vi "Mes Remote Telephone.vi"(8 "error in (no error)":errorcluster, 11 "Main":T1={"Tite"="", "Base path"=path "", "Table"=[], "Stations"=[], "Shield Array"=[], "UPHs"=[], "VISA"={"VISA"="", "baud rate"=9600, "data bits"=8, "parity"=enum."None", "stop bits"=10, "flow control"=0}, "Path"={"roof"=path "", "Config"=path "", "Png"=path ""}, "Ctr"={"DB Dispaly"=refnum, "Error Table"=refnum, "Display"=refnum, "Login"=refnum, "Exit"=refnum, "FTT_Submit"=refnum}, "Login"={"User"="", "Grade"=""}, "information"={"cause"="", "Type"=enum."Inform", "code"=0, "Suroce"="", "Status"=FALSE}, "Local DB"={"Connstr"="", "Database"={"Constr"={"Driver"="", "Server"="", "User"="", "Pwd"="", "Database"=""}, "conn ref"=refnum, "State"=FALSE}}, "Remote DB"={"Connstr"="", "Database"={"Constr"={"Driver"="", "Server"="", "User"="", "Pwd"="", "Database"=""}, "conn ref"=refnum, "State"=FALSE}}, "FTT TV"="", "ExchangeTime"=0, "NVH"="", "EOL Path"=path ""} {"VISA"."flow control" items=["None", "XON/XOFF", "RTS/CTS", "XON/XOFF & RTS/CTS", "DTR/DSR", "XON/XOFF & DTR/DSR"]; "VISA"."stop bits" items=["1.0"=10, "1.5"=15, "2.0"=20]}) -> (0 "error out":errorcluster)   [LabVIEW 2014]
uses:
  Type'def/Mes Table.ctl
  <vilib>/ptbypt/NI_PtbyPt.lvlib
  Type'def/UPH Config.ctl
  VISA/Ctr/VISA Ctr.ctl
  Type'def/Main Ctr Ref.ctl
  Type'def/User Login.ctl
  Database/Ctr/Constr.ctl
  <vilib>/addons/database/Connection.llb/Conn ObjectReference.ctl
  <vilib>/addons/database/NI_Database_API.lvlib
  Database/Ctr/Conneect State.ctl
  Type'def/MainCtr.ctl
panel:
  in  "x 2":bool
  out "数组":i32[](array[numeric])
  in  "x":bool
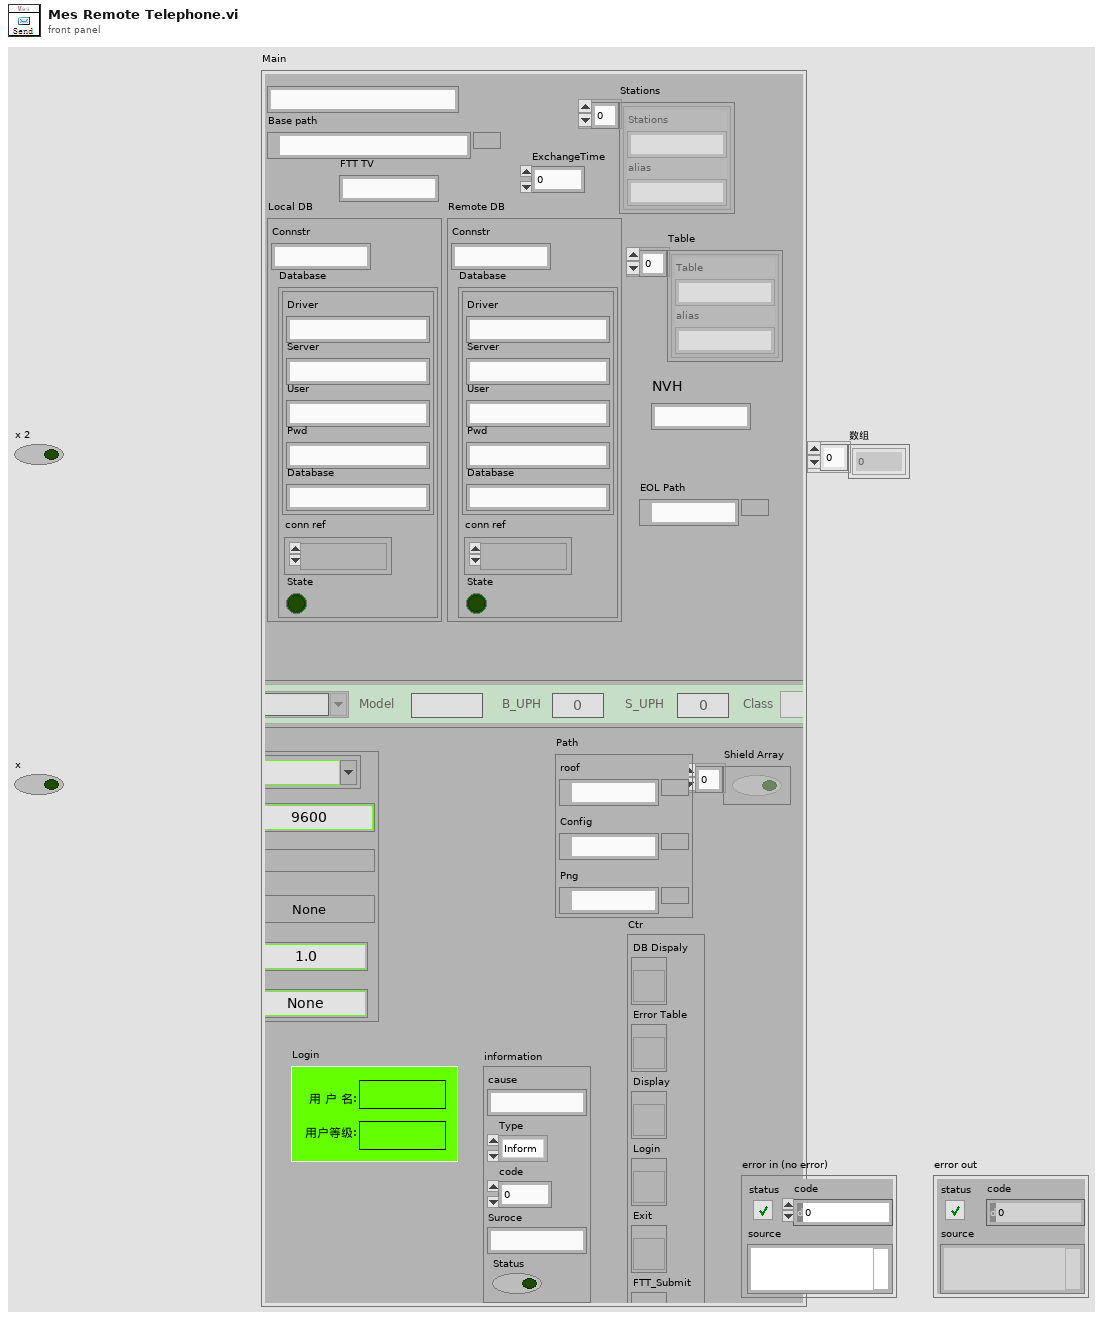
[diagram p1: front panel]
types:
  T1 = typedef "MainCtr.ctl" = cluster{"Tite":string, "Base path":path, "Table":cluster{"Table":string, "alias":string}[], "Stations":cluster{"Stations":string, "alias":string}[], "Shield Array":bool[], "UPHs":T2[], "VISA":T3, "Path":cluster{"roof":path, "Config":path, "Png":path}, "Ctr":T4, "Login":T5, "information":cluster{"cause":string, "Type":enum16{"Inform", "Warning", "Alarm"}, "code":i32, "Suroce":string, "Status":bool}, "Local DB":cluster{"Connstr":string, "Database":T6}, "Remote DB":cluster{"Connstr":string, "Database":T6}, "FTT TV":string, "ExchangeTime":i32, "NVH":string, "EOL Path":path}
  T2 = typedef "UPH Config.ctl" = cluster{"Line_No":string, "Model":string, "B_UPH ":i16, "S_UPH  ":i16, "Class":enum16{"Big", "Small"}}
  T3 = typedef "VISA Ctr.ctl" = cluster{"VISA":refnum<visa-resource-name>, "baud rate":u32, "data bits":u16, "parity":enum16{"None", "Odd", "Even", "Mark", "Space"}, "stop bits":u16, "flow control":u16}
  T4 = typedef "Main Ctr Ref.ctl" = cluster{"DB Dispaly":refnum<vi>, "Error Table":refnum<vi>, "Display":refnum<vi>, "Login":refnum<vi>, "Exit":refnum<vi>, "FTT_Submit":refnum<vi>}
  T5 = typedef "User Login.ctl" = cluster{"User":string, "Grade":string}
  T6 = typedef "Conneect State.ctl" = cluster{"Constr":T7, "conn ref":T8, "State":bool}
  T7 = typedef "Constr.ctl" = cluster{"Driver":string, "Server":string, "User":string, "Pwd":string, "Database":string}
  T8 = typedef "NI_Database_API.lvlib/Conn ObjectReference.ctl" = refnum<k1>
  T9 = cluster{"Model":string, "Actual":string, "NG":string}
  T10 = cluster{"cause":string, "Type":enum16{"Inform", "Warning", "Alarm"}, "code":i32, "Suroce":string, "Status":bool}
  T11 = typedef "Mes Table.ctl" = cluster{"DateInfo":timestamp, "Shift":string, "Line_Name":string, "ProjectName":string, "AvaType":string, "AvaValue":string, "Remark":string}
  T12 = cluster{"Outline_Type":string[], "Mess FTT":cluster{"Model":string, "Actual":string, "NG":string}, "Model":string[], "Main ":T1, "mes":T11, "information":cluster{"cause":string, "Type":enum16{"Inform", "Warning", "Alarm"}, "code":i32, "Suroce":string, "Status":bool}, "Insert/Update(Run)":bool[], "CT":string, "Mode":enum16{"Eight", "EModel", "Outline"}, "Insert/Update(History)":bool[]}
  T13 = typedef "FTT Display Type.ctl" = cluster{"Line.No":string, "Model":string, "Color":string, "UPH":dbl, "Plan":dbl, "Target Rate":dbl, "Target ":dbl, "Actual":dbl, "FTT":dbl, "FTT Rate":dbl, "Repaired":dbl, "Reject":dbl, "Ouline":dbl, "Line State":string}
  T14 = cluster{"Display":T13, "Class":enum16{"Big", "Small"}}
  T15 = typedef "Phone Var.ctl" = cluster{"Mes":bool, "Model":string}
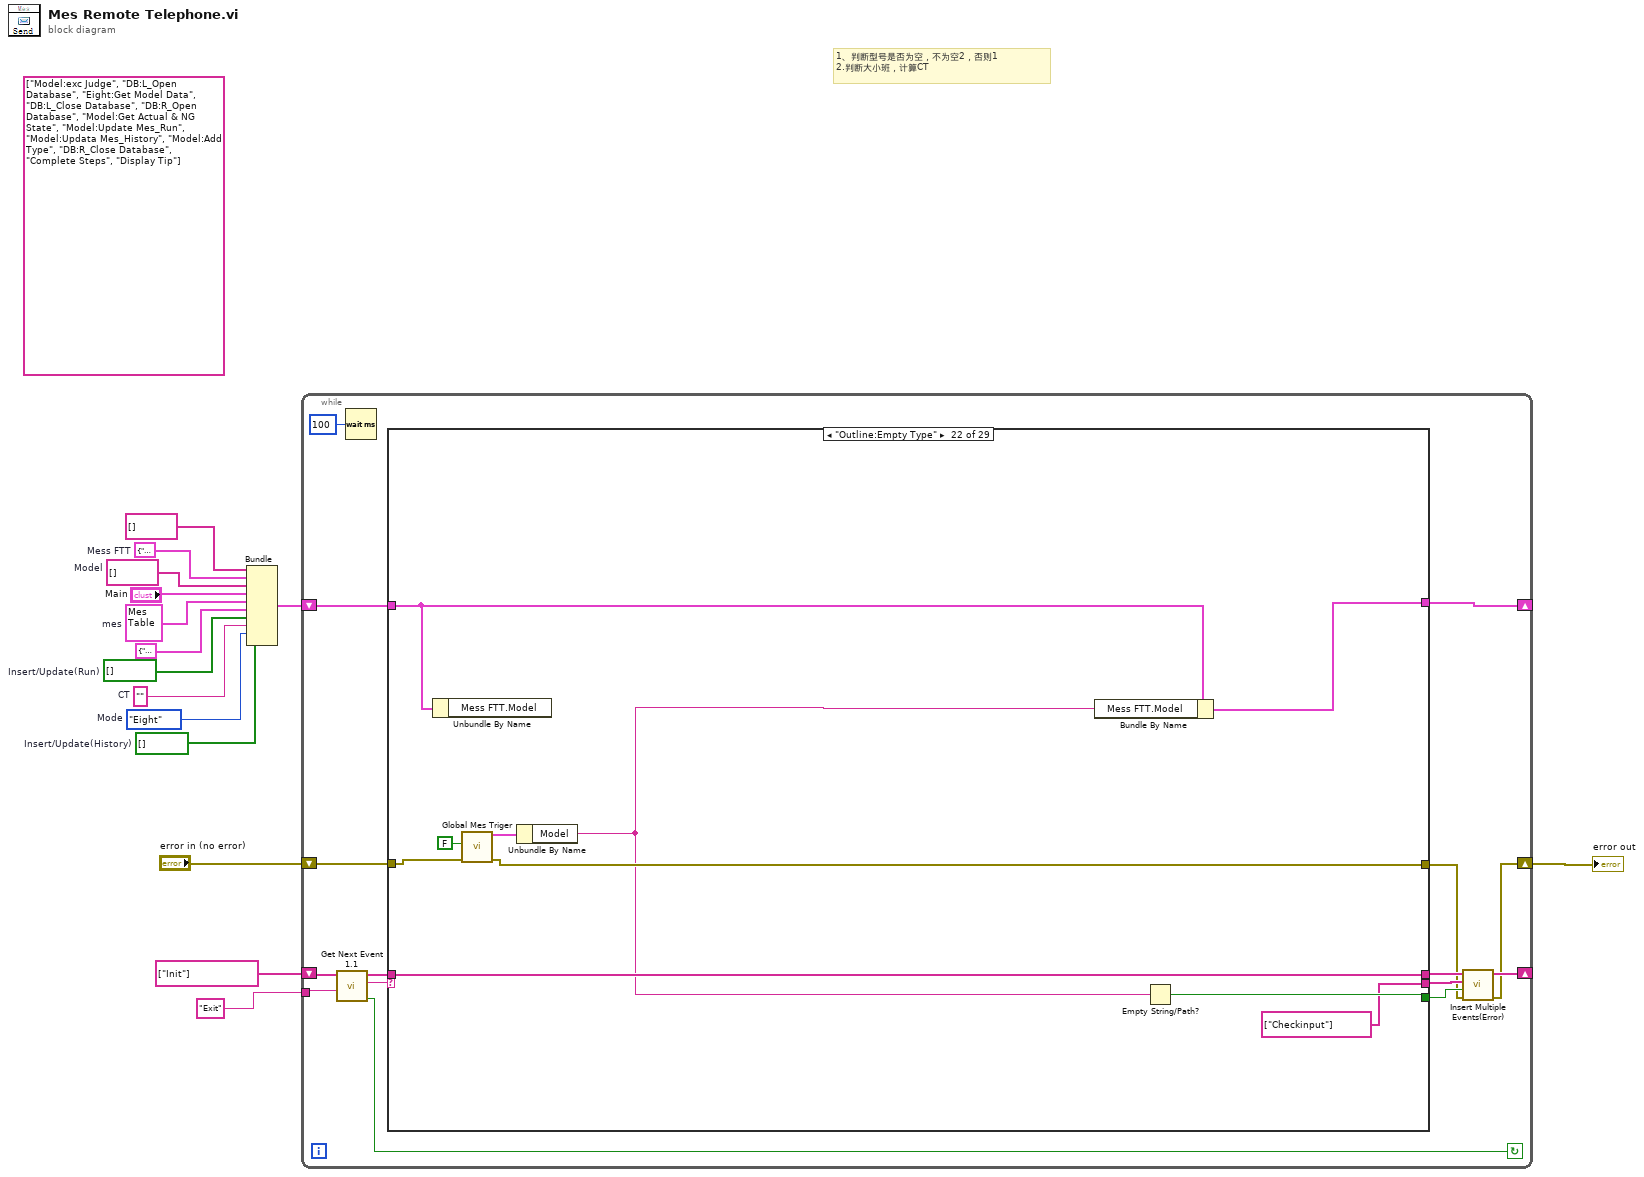
[diagram p0: block diagram]
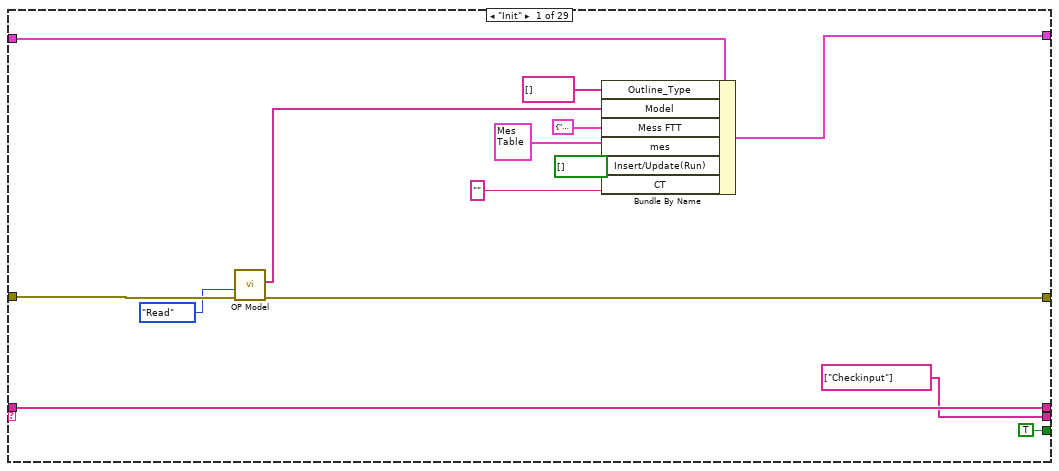
[diagram p2: hidden frame]
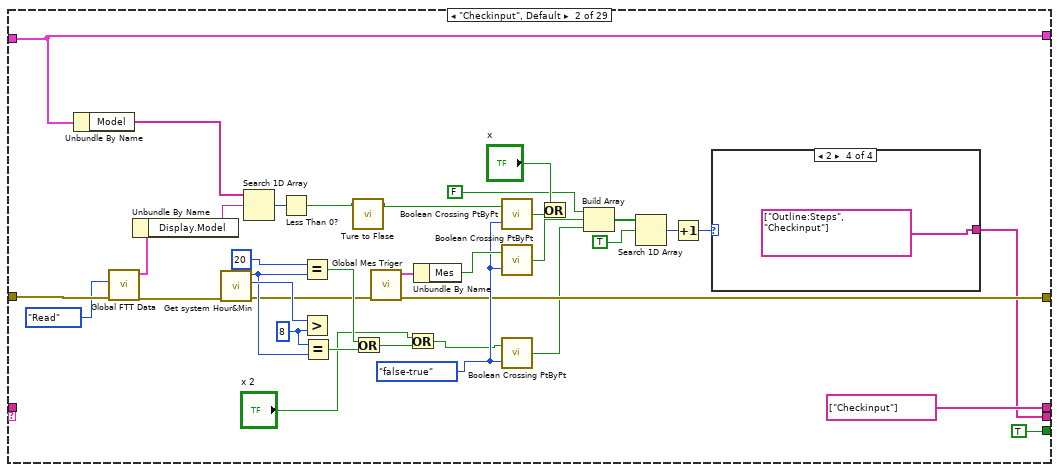
[diagram p3: hidden frame]
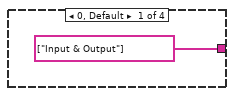
[diagram p4: hidden frame]
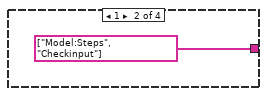
[diagram p5: hidden frame]
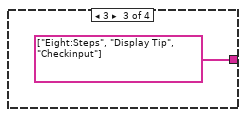
[diagram p6: hidden frame]
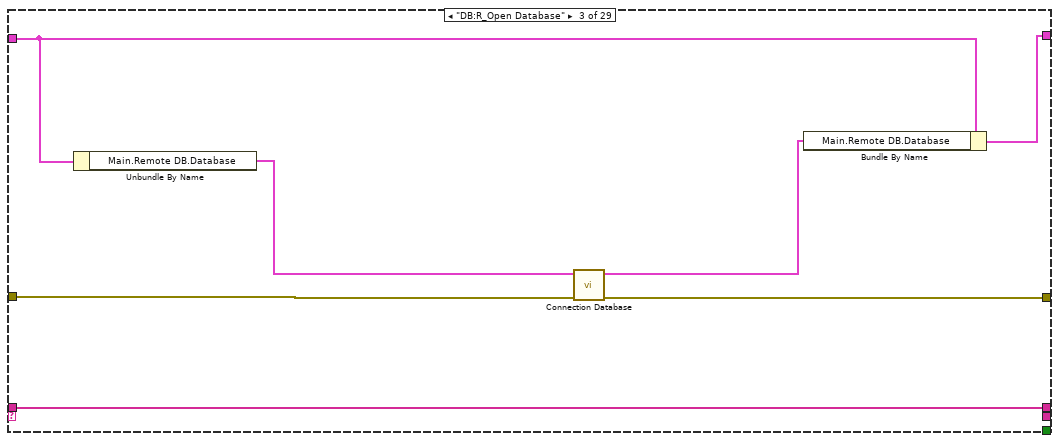
[diagram p7: hidden frame]
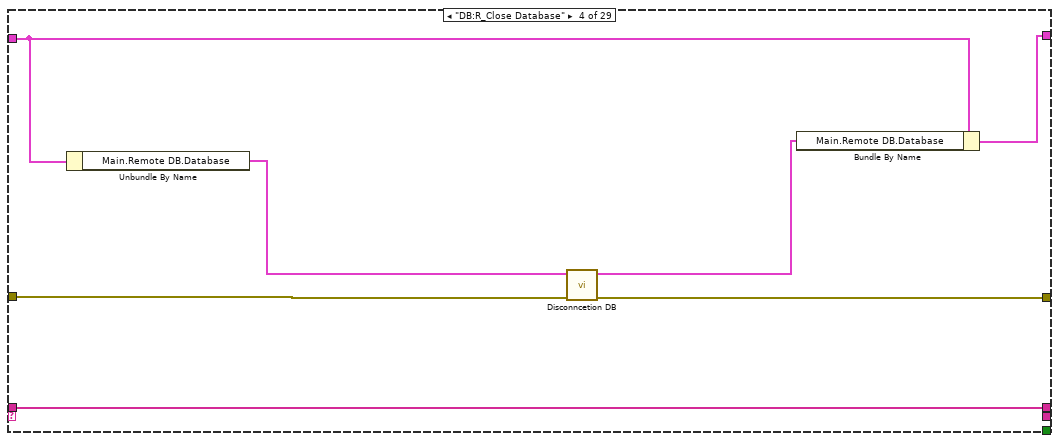
[diagram p8: hidden frame]
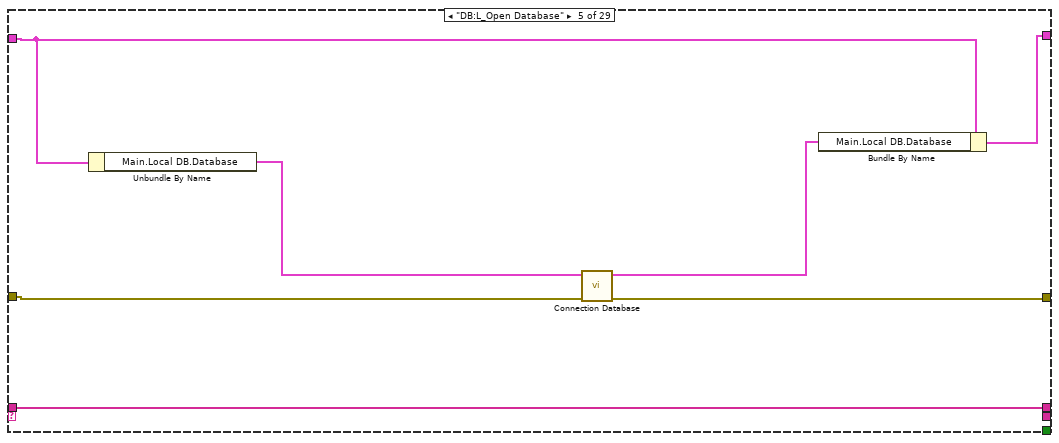
[diagram p9: hidden frame]
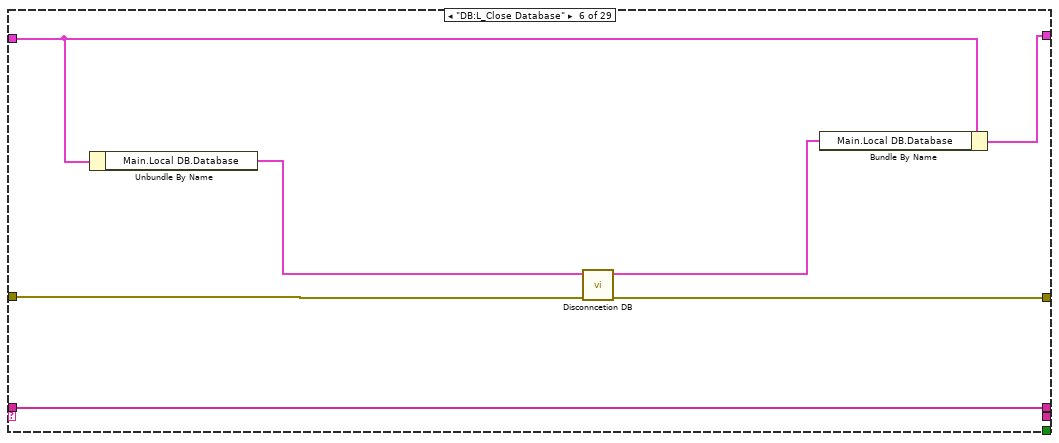
[diagram p10: hidden frame]
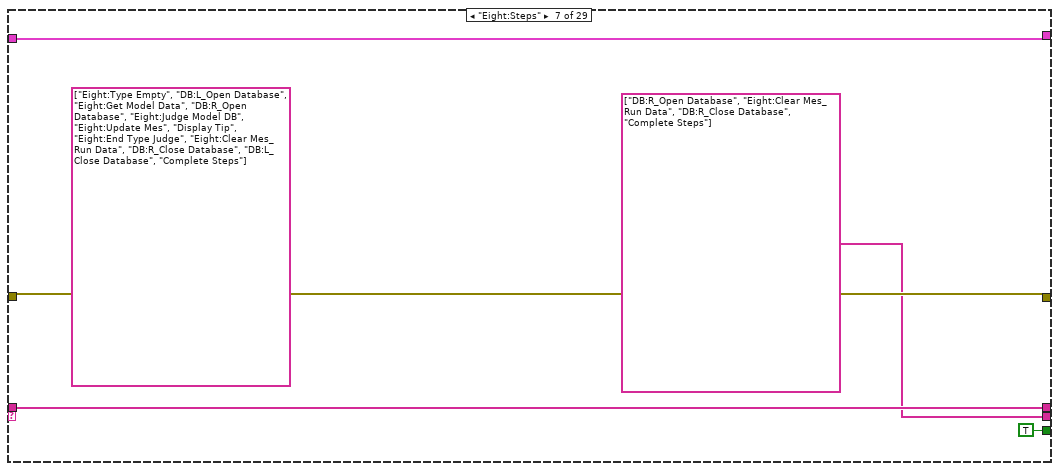
[diagram p11: hidden frame]
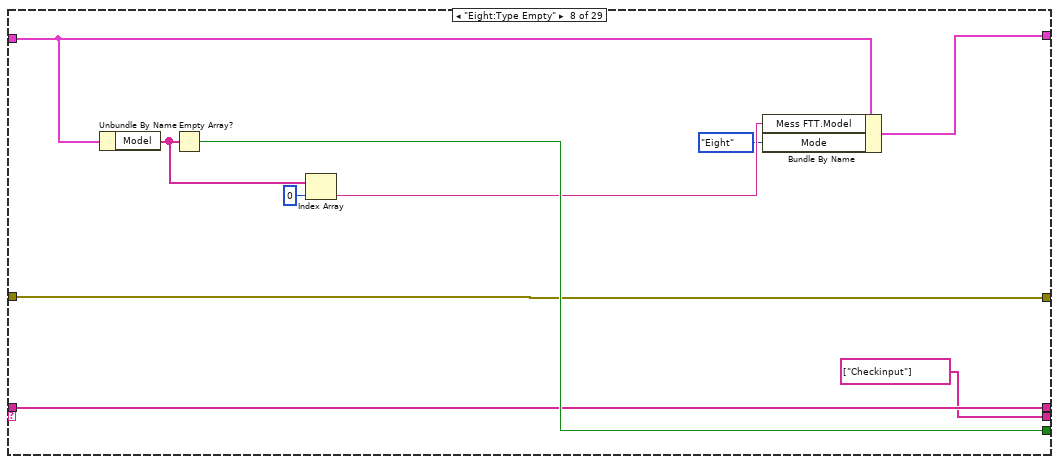
[diagram p12: hidden frame]
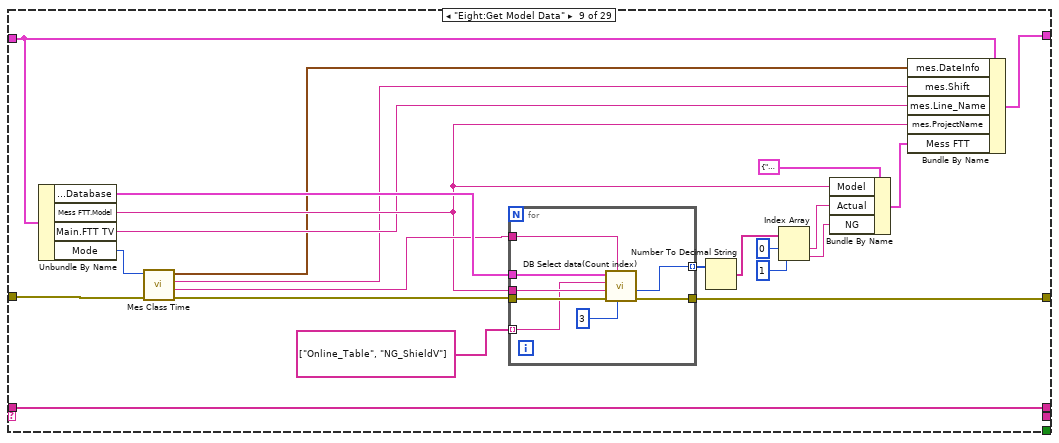
[diagram p13: hidden frame]
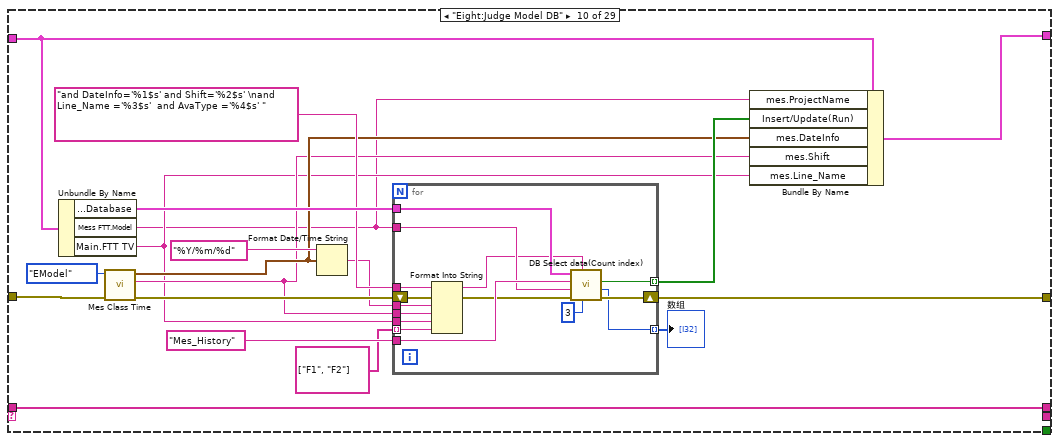
[diagram p14: hidden frame]
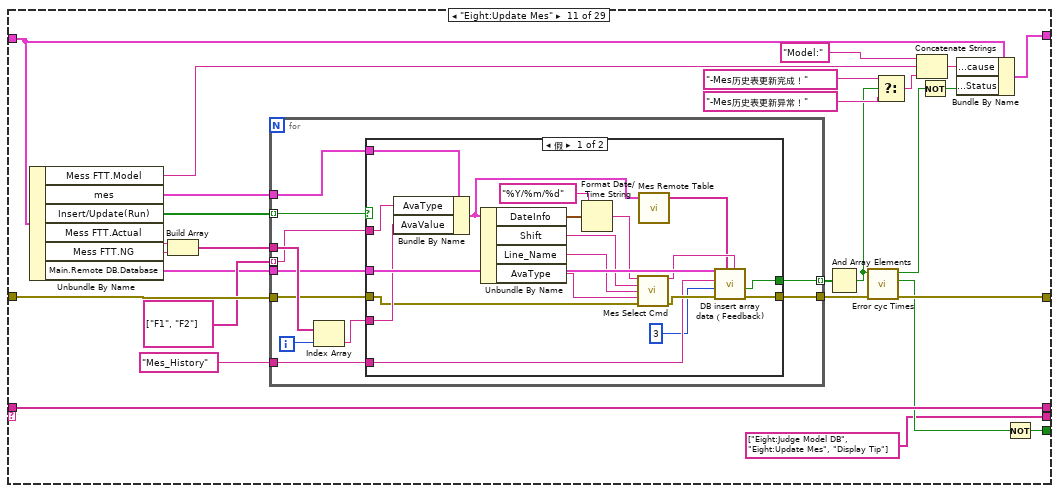
[diagram p15: hidden frame]
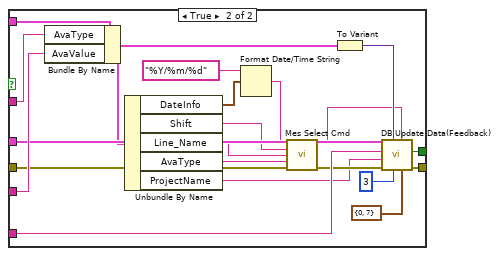
[diagram p16: hidden frame]
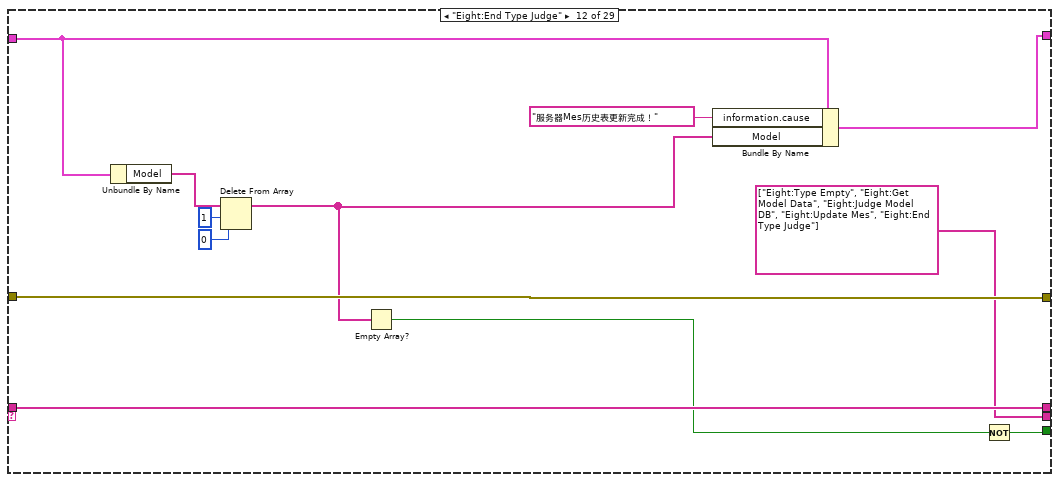
[diagram p17: hidden frame]
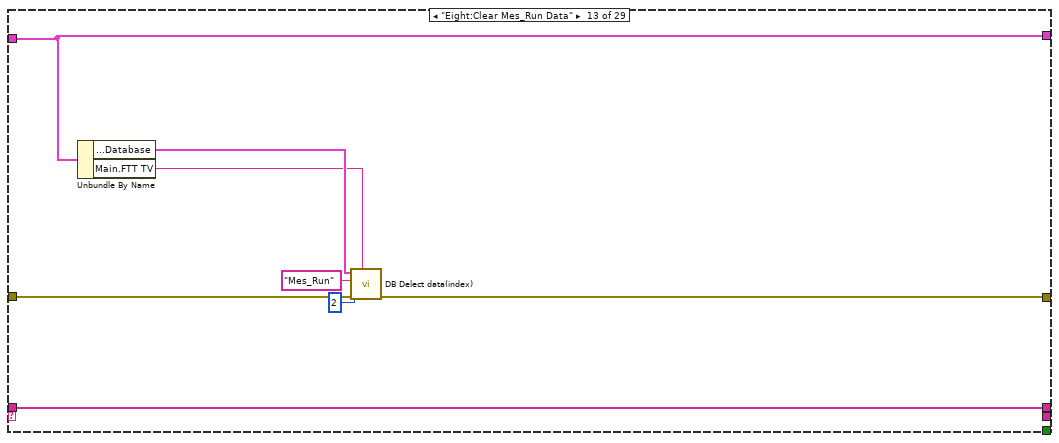
[diagram p18: hidden frame]
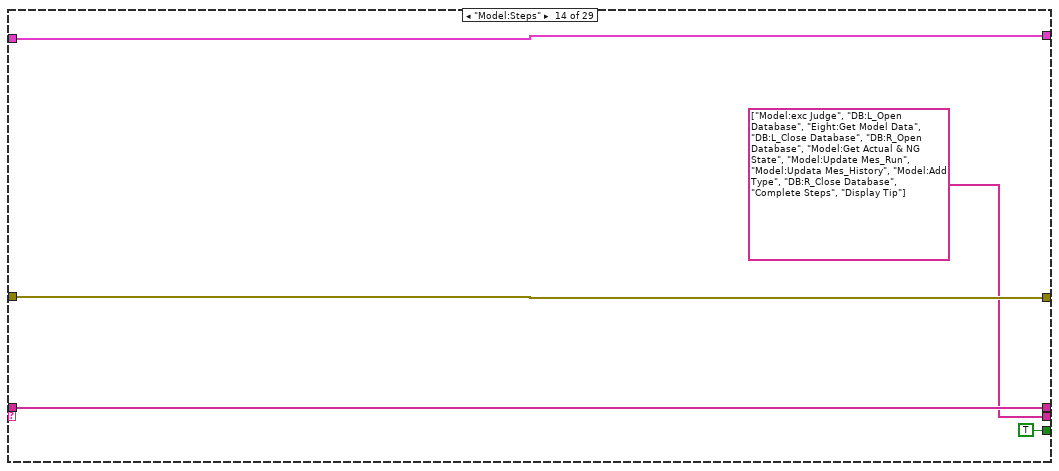
[diagram p19: hidden frame]
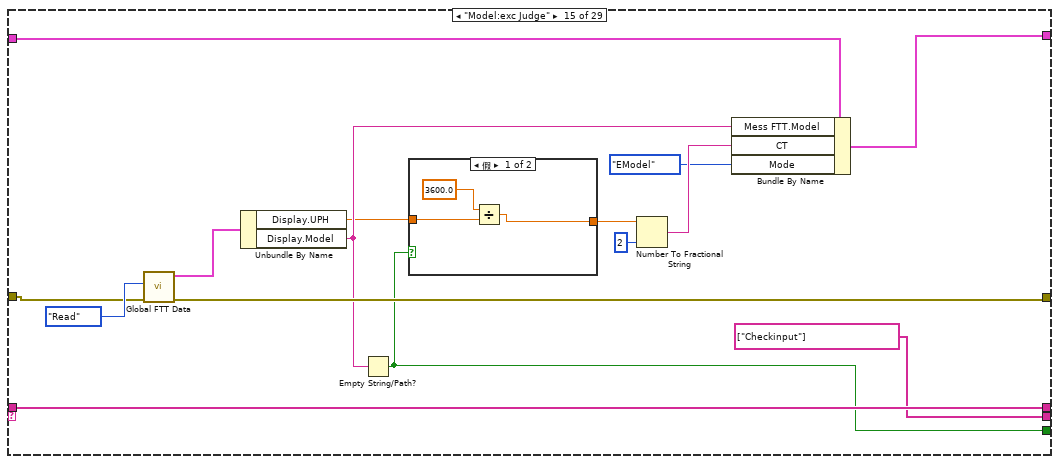
[diagram p20: hidden frame]
diagram:
  w1 = bool[] []  # Insert/Update(History)
  (unwired) string[] ["Model:exc Judge", "DB:L_Open Database", "Eight:Get Model Data", "DB:L_Close Database", "DB:R_Open Database", "Model:Get Actual & NG State", "Model:Update Mes_Run", "Model:Updata Mes_History", "Model:Add Type", "DB:R_Close Database", "Complete Steps", "Display Tip"]
  w2 = enum16{"Eight", "EModel", "Outline"}."Eight"  # Mode
  w3 = ""  # CT
  w5 = bool[] []  # Insert/Update(Run)
  w6 = T9 {"Model"="", "Actual"="", "NG"=""}  # Mess FTT
  w7 = string[] []  # Model
  w10 = T11 {"DateInfo"=timestamp(0 s since 1904-01-01), "Shift"="", "Line_Name"="", "ProjectName"="", "AvaType"="", "AvaValue"="", "Remark"=""}  # mes
  # "1、判断型号是否为空，不为空2，否则1\n2.判断大小班，计算CT"
  n1 = Bundle("Outline_Type"=string[] [], "Mess FTT"=w6, "Model"=w7, "Main"="Main", "mes"=w10, "information"=T10 {"cause"="", "Type"=enum."Inform", "code"=0, "Suroce"="", "Status"=FALSE}, "Insert/Update(Run)"=w5, "CT"=w3, "Mode"=w2, "Insert/Update(History)"=w1) -> (w12:T12)  [unwired: 1 in]
  n2 = while {
    tunnel: "Exit" ("Exit Event") -> [w27]
    shift-right: [w23] -> _
    shift-left: string[] ["Init"] -> [w28]
    shift-right: [w16] -> w9
    shift-left: "error in (no error)" -> [w26]
    shift-right: [w19] -> _
    shift-left: w12 -> [w24]
    stop <- w29 continue-if-true
    n3 = call "Get Next Event 1.1.vi"("Exit Event"=w27, "event queue in"=w28) -> ("Condition (Exit:F)"=w29:bool, "next event"=w30:string, "event queue out"=w25:string[])  [unwired: 6 in, 1 out]
    n4 = Wait (ms)(milliseconds to wait=u32 100) -> ()  [unwired: 1 out]
    n5 = case shown="\"Outline:Empty Type\"" w30 {
      tunnel: w26 -> [w34 w78 w89 w97 w103 w110 w114 w126 w135 w173 w217 w276 w288 w293 w308 w324 w349 w391 w463 w542 w561 w572 w585 w668 w673 w680 w686 w689 w697]
      tunnel: w25 -> [w44 _ w85 w98 w100 w106 w116 w125 w149 w176 w218 w275 w282 w292 w306 w322 w346 w389 w485 w553 w567 w577 w583 w661 w672 w681 w685 w692 w700]
      tunnel: w24 -> [w35 w60 w87 w94 w102 w109 w117 w123 w138 w165 w203 w278 w289 w294 w305 w321 w350 w388 w462 w552 w565 w574 w584 w663 w675 w682 w687 w693 w704]
      tunnel: [w33 w61 w86 w96 w101 w107 w114 w126 w146 w168 w206 w276 w283 w293 w307 w323 w348 w390 w483 w541 w559 w571 w582 w668 w673 w676 w686 w694 w705] -> w17
      tunnel: [w44 string[] ["Checkinput"] w85 w98 w100 w106 w116 w125 w149 w176 w218 w275 w282 w292 w306 w322 w346 w389 w485 w553 w567 w577 w583 w661 w672 w681 w685 w692 w700] -> w22
      tunnel: [TRUE ("Insert all? (T)") TRUE ("Insert all? (T)") _ _ _ _ TRUE ("Insert all? (T)") w127 _ _ w205 w273 _ TRUE ("Insert all? (T)") w300 _ _ w385 w484 _ TRUE ("Insert all? (T)") w576 w579 w658 _ w678 TRUE ("Insert all? (T)") _ TRUE ("Insert all? (T)")] -> w21
      tunnel: [string[] ["Checkinput"] w53 _ _ _ _ string[] ["DB:R_Open Database", "Eight:Clear Mes_Run Data", "DB:R_Close Database", "Complete Steps"] string[] ["Checkinput"] _ _ string[] ["Eight:Judge Model DB", "Eight:Update Mes", "Display Tip"] string[] ["Eight:Type Empty", "Eight:Get Model Data", "Eight:Judge Model DB", "Eight:Update Mes", "Eight:End Type Judge"] _ string[] ["Model:exc Judge", "DB:L_Open Database", "Eight:Get Model Data", "DB:L_Close Database", "DB:R_Open Database", "Model:Get Actual & NG State", "Model:Update Mes_Run", "Model:Updata Mes_History", "Model:Add Type", "DB:R_Close Database", "Complete Steps", "Display Tip"] string[] ["Checkinput"] _ _ w378 w475 _ string[] ["Model:exc Judge", "Outline:Empty Type", "DB:L_Open Database", "Eight:Get Model Data", "DB:R_Open Database", "Model:Get Actual & NG State(Run)", "Model:Get Actual & NG State(History)", "Model:Update Mes_Run", "Model:Updata Mes_History", "DB:L_Close Database", "DB:R_Close Database", "Display Tip "] string[] ["Checkinput"] string[] ["Outline:Mes_Run Update"] string[] ["Outline:Empty Type", "Eight:Get Model Data", "Outline:Mes_Run Update", "Outline:End Type Judge"] _ string[] ["Quit"] string[] ["Exit"] _ string[] ["Checkinput"]] -> w20
      tunnel: [w36 w60 w88 w93 w99 w108 w117 w122 w137 w164 w202 w277 w289 w294 w304 w320 w347 w387 w480 w551 w564 w573 w586 w662 w674 w682 w687 w693 w704] -> w19
      frame "Init" {
        n6 = call "OP Model.vi"("error in (no error)"=w34, "Enum"=enum16{"init", "Read", "Write"}."Read") -> ("error out"=w33:errorcluster, "ArrayStr out"=w31:string[])  [unwired: 7 in, 1 out]
        n7 = Bundle By Name(cluster=w35, "Outline_Type"=string[] [], "Model"=w31, "Mess FTT"=T9 {"Model"="", "Actual"="", "NG"=""}, "mes"=T11 {"DateInfo"=timestamp(0 s since 1904-01-01), "Shift"="", "Line_Name"="", "ProjectName"="", "AvaType"="", "AvaValue"="", "Remark"=""}, "Insert/Update(Run)"=bool[] [] ("Insert/Update"), "CT"="") -> (w36:T12)
      }
      frame "Checkinput", Default {
        w62 = enum16{"either", "false-true", "true-false"}."false-true" ("direction")
        w70 = 8 ("y")
        n8 = Unbundle By Name(w60) -> ("Model"=w74:string[])
        n9 = call "Global FTT Data.vi"("error in (no error)"=w78, "Mode"=enum16{"Read", "Write"}."Read") -> ("error out"=w72:errorcluster, "Cluster"=w76:T14)  [unwired: 8 in]
        n10 = Unbundle By Name(w76) -> ("Display.Model"=w75:string)
        n11 = call "Get system Hour&Min.vi"("error in (no error)"=w72) -> ("error out"=w65:errorcluster, "minute"=w69:i32, "hour"=w68:i32)  [unwired: 7 in, 1 out]
        n12 = Search 1D Array(1D array=w74, element=w75) -> (index of element=w73:i32)  [unwired: 1 in]
        n13 = Less Than 0?(x=w73) -> (x < 0?=w50:bool)
        n14 = Equal?(x=20, y=w68) -> (x = y?=w66:bool)
        n15 = Greater?(x=w69, y=w70) -> ()  [unwired: 1 out]
        n16 = Equal?(x=w70, y=w68) -> (x = y?=w67:bool)
        n17 = call "Ture to Flase.vi"("in"=w50) -> ("Out"=w49:bool)  [unwired: 4 in]
        n18 = Or(x=w66, y=w67) -> (x .or. y?=w48:bool)
        n19 = call "Global Mes Triger.vi"("error in (no error)"=w65) -> ("error out"=w61:errorcluster, "Var out"=w64:T15)  [unwired: 9 in]
        n20 = Or(x="x 2", y=w48) -> (x .or. y?=w47:bool)
        n21 = Unbundle By Name(w64) -> ("Mes"=w63:bool)
        n22 = call <vilib>:"Boolean Crossing PtByPt.vi"("direction"=w62, "input"=w49) -> ("crossing"=w52:bool)  [unwired: 1 in]
        n23 = call <vilib>:"Boolean Crossing PtByPt.vi"("direction"=w62, "input"=w63) -> ("crossing"=w59:bool)  [unwired: 1 in]
        n24 = call <vilib>:"Boolean Crossing PtByPt.vi"("direction"=w62, "input"=w47) -> ("crossing"=w58:bool)  [unwired: 1 in]
        n25 = Or(x="x", y=w52) -> ()  [unwired: 1 out]
        n26 = Build Array(FALSE ("element"), w59, w58) -> (w57:bool[])
        n27 = Search 1D Array(1D array=w57, element=TRUE) -> (index of element=w55:i32)  [unwired: 1 in]
        n28 = Increment(x=w55) -> (x+1=w54:i32)
        n29 = case shown="2" w54 {
          tunnel: [string[] ["Input & Output"] string[] ["Model:Steps", "Checkinput"] string[] ["Eight:Steps", "Display Tip", "Checkinput"] string[] ["Outline:Steps", "Checkinput"]] -> w53
          frame 0, Default {
          }
          frame 1 {
          }
          frame 3 {
          }
          frame 2 {
          }
        }
      }
      frame "DB:R_Open Database" {
        n30 = Unbundle By Name(w87) -> ("Main.Remote DB.Database"=w91:T6)
        n31 = call "Connection Database.vi"("error in (no error)"=w89, "Connncet State"=w91) -> ("error out"=w86:errorcluster, "Connncet State out"=w90:T6)  [unwired: 8 in]
        n32 = Bundle By Name(cluster=w87, "Main.Remote DB.Database"=w90) -> (w88:T12)
      }
      frame "DB:R_Close Database" {
        n33 = Unbundle By Name(w94) -> ("Main.Remote DB.Database"=w95:T6)
        n34 = call "Disconncetion DB.vi"("error in (no error)"=w97, "Connncet State"=w95) -> ("error out"=w96:errorcluster, "Connect State"=w92:T6)  [unwired: 8 in]
        n35 = Bundle By Name(cluster=w94, "Main.Remote DB.Database"=w92) -> (w93:T12)
      }
      frame "DB:L_Open Database" {
        n36 = Unbundle By Name(w102) -> ("Main.Local DB.Database"=w105:T6)
        n37 = call "Connection Database.vi"("error in (no error)"=w103, "Connncet State"=w105) -> ("error out"=w101:errorcluster, "Connncet State out"=w104:T6)  [unwired: 8 in]
        n38 = Bundle By Name(cluster=w102, "Main.Local DB.Database"=w104) -> (w99:T12)
      }
      frame "DB:L_Close Database" {
        n39 = Unbundle By Name(w109) -> ("Main.Local DB.Database"=w112:T6)
        n40 = call "Disconncetion DB.vi"("error in (no error)"=w110, "Connncet State"=w112) -> ("error out"=w107:errorcluster, "Connect State"=w111:T6)  [unwired: 8 in]
        n41 = Bundle By Name(cluster=w109, "Main.Local DB.Database"=w111) -> (w108:T12)
      }
      frame "Eight:Steps" {
        (unwired) string[] ["Eight:Type Empty", "DB:L_Open Database", "Eight:Get Model Data", "DB:R_Open Database", "Eight:Judge Model DB", "Eight:Update Mes", "Display Tip", "Eight:End Type Judge", "Eight:Clear Mes_Run Data", "DB:R_Close Database", "DB:L_Close Database", "Complete Steps"]
      }
      frame "Eight:Type Empty" {
        n42 = Unbundle By Name(w123) -> ("Model"=w121:string[])
        n43 = Empty Array?(array=w121) -> (empty?=w127:bool)
        n44 = Index Array(array=w121, index=0 ("索引")) -> (element=w119:string)
        n45 = Bundle By Name(cluster=w123, "Mess FTT.Model"=w119, "Mode"=enum16{"Eight", "EModel", "Outline"}."Eight") -> (w122:T12)
      }
      frame "Eight:Get Model Data" {
        n46 = Unbundle By Name(w138) -> ("Main.Local DB.Database"=w148:T6, "Mess FTT.Model"=w132:string, "Main.FTT TV"=w131:string, "Mode"=w128:enum16{"Eight", "EModel", "Outline"})
        n47 = call "Mes Class Time.vi"("error in (no error)"=w135, "Mode"=w128) -> ("error out"=w134:errorcluster, "结果字符串"=w133:string, "Class"=w130:string, "s? t:f"=w129:timestamp)  [unwired: 6 in]
        n48 = for {
          tunnel: w134 -> [w157]
          tunnel: w148 -> [w156]
          tunnel: w132 -> [w155]
          tunnel: string[] ["Online_Table", "NG_ShieldV"] -> [w153] mode=indexing
          tunnel: [w152] -> w146
          tunnel: [w151] -> w144 mode=indexing
          tunnel: w133 -> [w150]
          n49 = call "DB Select data(Count index).vi"("index"=3, "Condtion"=w150, "error in (no error)"=w157, "Code"=w155, "Tabe"=w153, "Connncet State"=w156) -> ("error out"=w152:errorcluster, "Count"=w151:i32)  [unwired: 2 in, 2 out]
        }
        n50 = Number To Decimal String(number=w144) -> (decimal integer string=w143:string[])  [unwired: 1 in]
        n51 = Index Array(array=w143, index #1=0 ("index"), index #2=1 ("index")) -> (element #1=w140:string, element #2=w139:string)
        n52 = Bundle By Name(cluster=T9 {"Model"="", "Actual"="", "NG"=""} ("Cluster"), "Model"=w132, "Actual"=w140, "NG"=w139) -> (w136:T9)
        n53 = Bundle By Name(cluster=w138, "mes.DateInfo"=w129, "mes.Shift"=w130, "mes.Line_Name"=w131, "mes.ProjectName"=w132, "Mess FTT"=w136) -> (w137:T12)
      }
      frame "Eight:Judge Model DB" {
        n54 = Unbundle By Name(w165) -> ("Main.Remote DB.Database"=w175:T6, "Mess FTT.Model"=w160:string, "Main.FTT TV"=w161:string)
        n55 = call "Mes Class Time.vi"("error in (no error)"=w173, "Mode"=enum16{"Eight", "EModel", "Outline"}."EModel") -> ("error out"=w172:errorcluster, "Class"=w162:string, "s? t:f"=w163:timestamp)  [unwired: 6 in, 1 out]
        n56 = Format Date/Time String(time format string (%c)="%Y/%m/%d", seconds (now)=w163) -> (date/time string=w169:string)  [unwired: 1 in]
        n57 = for {
          tunnel: w175 -> [w191]
          tunnel: "Mes_History" -> [w190]
          tunnel: w160 -> [w189]
          tunnel: "and DateInfo='%1$s' and Shift='%2$s' \nand Line_Name ='%3$s'  and AvaType ='%4$s' " -> [w185]
          tunnel: w169 -> [w184]
          tunnel: w162 -> [w183]
          tunnel: w161 -> [w182]
          tunnel: [w179] -> w166 mode=indexing
          shift-right: [w181] -> w168
          shift-left: w172 -> [w187]
          tunnel: string[] ["F1", "F2"] -> [w178] mode=indexing
          tunnel: [w177] -> w159 mode=indexing
          n58 = Format Into String(format string=w185, error in=w187, w184, w183, w182, w178) -> (resulting string=w180:string, error out=w186:errorcluster)  [unwired: 1 in]
          n59 = call "DB Select data(Count index).vi"("index"=3, "Condtion"=w180, "error in (no error)"=w186, "Code"=w189, "Tabe"=w190, "Connncet State"=w191) -> ("error out"=w181:errorcluster, "Count"=w177:i32, "state"=w179:bool)  [unwired: 2 in, 1 out]
        }
        "数组" <- w159
        n60 = Bundle By Name(cluster=w165, "mes.ProjectName"=w160, "Insert/Update(Run)"=w166, "mes.DateInfo"=w163, "mes.Shift"=w162, "mes.Line_Name"=w161) -> (w164:T12)
      }
      frame "Eight:Update Mes" {
        n61 = Unbundle By Name(w203) -> ("Mess FTT.Model"=w197:string, "mes"=w211:T11, "Insert/Update(Run)"=w216:bool[], "Mess FTT.Actual"=w215:string, "Mess FTT.NG"=w214:string, "Main.Remote DB.Database"=w210:T6)
        n62 = Build Array(w215, w214) -> (w213:string[])
        n63 = for {
          tunnel: w217 -> [w223]
          tunnel: w216 -> [w227] mode=indexing
          tunnel: w213 -> [w228]
          tunnel: string[] ["F1", "F2"] -> [w224] mode=indexing
          tunnel: w211 -> [w225]
          tunnel: w210 -> [w222]
          tunnel: "Mes_History" -> [w221]
          tunnel: [w220] -> w207
          tunnel: [w219] -> w208 mode=indexing
          i -> [w229]
          n64 = Index Array(array=w228, index=w229) -> (element=w226:string)
          n65 = case shown="假" w227 {
            tunnel: w226 -> [w244 w267]
            tunnel: w225 -> [w246 w269]
            tunnel: w224 -> [w245 w268]
            tunnel: w223 -> [w243 w264]
            tunnel: w222 -> [w247 w266]
            tunnel: w221 -> [w241 w265]
            tunnel: [w248 w253] -> w220
            tunnel: [w232 w252] -> w219
            frame False {
              n66 = Bundle By Name(cluster=w246, "AvaType"=w245, "AvaValue"=w244) -> (w231:T11)
              n67 = Unbundle By Name(w231) -> ("DateInfo"=w238:timestamp, "Shift"=w235:string, "Line_Name"=w234:string, "AvaType"=w233:string)
              n68 = Format Date/Time String(time format string (%c)="%Y/%m/%d", seconds (now)=w238) -> (date/time string=w236:string)  [unwired: 1 in]
              n69 = call "Mes Select Cmd.vi"("DateInfo"=w236, "Shift"=w235, "Line_Name"=w234, "AvaType"=w233, "error in (no error)"=w243) -> ("resulting string"=w239:string, "error out"=w242:errorcluster)  [unwired: 9 in]
              n70 = call "Mes Remote Table.vi"("mes"=w231) -> ("appended array"=w230:string[])  [unwired: 4 in]
              n71 = call "DB insert array data（Feedback).vi"("Condtion"=w239, "Data"=w230, "error in (no error)"=w242, "index"=3, "table"=w241, "Connncet State"=w247) -> ("error out"=w248:errorcluster, "state"=w232:bool)  [unwired: 3 in, 1 out]
            }
            frame True {
              n72 = Bundle By Name(cluster=w269, "AvaType"=w268, "AvaValue"=w267) -> (w262:T11)
              n73 = Unbundle By Name(w262) -> ("DateInfo"=w259:timestamp, "Shift"=w257:string, "Line_Name"=w256:string, "AvaType"=w255:string, "ProjectName"=w254:string)
              n74 = Format Date/Time String(time format string (%c)="%Y/%m/%d", seconds (now)=w259) -> (date/time string=w258:string)  [unwired: 1 in]
              n75 = call "Mes Select Cmd.vi"("DateInfo"=w258, "Shift"=w257, "Line_Name"=w256, "AvaType"=w255, "error in (no error)"=w264) -> ("resulting string"=w251:string, "error out"=w263:errorcluster)  [unwired: 9 in]
              n76 = To Variant(anything=w262) -> (Variant=w261:variant)
              n77 = call "DB Update Data(Feedback).vi"("Pos"=cluster{"index":i32, "Len":i32} {"index"=0, "Len"=7}, "condtinal"=w251, "Sel index"=3, "data"=w261, "error in (no error)"=w263, "Code"=w254, "table"=w265, "Connncet State"=w266) -> ("error out"=w253:errorcluster, "State"=w252:bool)  [unwired: 1 in, 1 out]
            }
          }
        }
        n78 = And Array Elements(Boolean array=w208) -> (logical AND=w193:bool)
        n79 = call "Error cyc Times.vi"("error in (no error)"=w207, "Status in"=w193) -> ("error out"=w206:errorcluster, "Cys Status"=w204:bool, "Status out"=w200:bool)  [unwired: 6 in, 1 out]
        n80 = Select(t="-Mes历史表更新完成！" ("string"), s=w193, f="-Mes历史表更新异常！" ("string")) -> (s? t:f=w192:string)
        n81 = Concatenate Strings("Model:" ("string"), w197, w192) -> (w199:string)
        n82 = Not(x=w200) -> (.not. x?=w201:bool)
        n83 = Bundle By Name(cluster=w203, "information.cause"=w199, "information.Status"=w201) -> (w202:T12)
        n84 = Not(x=w204) -> (.not. x?=w205:bool)
      }
      frame "Eight:End Type Judge" {
        n85 = Unbundle By Name(w278) -> ("Model"=w281:string[])
        n86 = Delete From Array(array=w281, length=1, index=0) -> (array with subset deleted=w274:string[])  [unwired: 1 out]
        n87 = Empty Array?(array=w274) -> (empty?=w272:bool)
        n88 = Bundle By Name(cluster=w278, "information.cause"="服务器Mes历史表更新完成！", "Model"=w274) -> (w277:T12)
        n89 = Not(x=w272) -> (.not. x?=w273:bool)
      }
      frame "Eight:Clear Mes_Run Data" {
        n90 = Unbundle By Name(w289) -> ("Main.Remote DB.Database"=w287:T6, "Main.FTT TV"=w286:string)
        n91 = call "DB Delect data(index).vi"("code"=w286, "error in (no error)"=w288, "index"=2, "table"="Mes_Run", "Connncet State"=w287) -> ("error out"=w283:errorcluster)  [unwired: 4 in, 2 out]
      }
      frame "Model:Steps" {
      }
      frame "Model:exc Judge" {
        n92 = call "Global FTT Data.vi"("error in (no error)"=w308, "Mode"=enum16{"Read", "Write"}."Read") -> ("error out"=w307:errorcluster, "Cluster"=w303:T14)  [unwired: 8 in]
        n93 = Unbundle By Name(w303) -> ("Display.UPH"=w299:dbl, "Display.Model"=w302:string)
        n94 = Empty String/Path?(string/path=w302) -> (empty?=w300:bool)
        n95 = case shown="假" w300 {
          tunnel: w299 -> [w311 _]
          tunnel: [w310 30.0 ("UPH")] -> w298
          frame False {
            n96 = Divide(x=3600.0, y=w311) -> (x/y=w310:dbl)
          }
          frame True {
          }
        }
        n97 = Number To Fractional String(number=w298, precision (6)=i16 2) -> (F-format string=w296:string)  [unwired: 2 in]
        n98 = Bundle By Name(cluster=w305, "Mess FTT.Model"=w302, "CT"=w296, "Mode"=enum16{"Eight", "EModel", "Outline"}."EModel") -> (w304:T12)
      }
      frame "Model:Get Actual & NG State(Run)" {
        n99 = Unbundle By Name(w321) -> ("Main.Remote DB.Database"=w330:T6, "Mess FTT.Model"=w316:string, "Main.FTT TV"=w317:string, "Mode"=w314:enum16{"Eight", "EModel", "Outline"})
        n100 = call "Mes Class Time.vi"("error in (no error)"=w324, "Mode"=w314) -> ("error out"=w328:errorcluster, "Class"=w318:string, "s? t:f"=w319:timestamp)  [unwired: 6 in, 1 out]
        n101 = Format Date/Time String(time format string (%c)="%Y/%m/%d", seconds (now)=w319) -> (date/time string=w326:string)  [unwired: 1 in]
        n102 = for {
          tunnel: w330 -> [w344]
          tunnel: "Mes_Run" -> [w343]
          tunnel: w316 -> [w342]
          tunnel: w326 -> [w337]
          tunnel: w318 -> [w336]
          tunnel: w317 -> [w335]
          tunnel: [w339] -> w315 mode=indexing
          shift-right: [w340] -> w323
          shift-left: w328 -> [w338]
          tunnel: string[] ["F1", "F2", "F3"] -> [w334] mode=indexing
          n103 = call "Mes Select Cmd.vi"("DateInfo"=w337, "h/r"=FALSE, "Shift"=w336, "Line_Name"=w335, "AvaType"=w334, "error in (no error)"=w338) -> ("resulting string"=w332:string, "error out"=w333:errorcluster)  [unwired: 8 in]
          n104 = call "DB Select data(Count index).vi"("index"=3, "Condtion"=w332, "error in (no error)"=w333, "Code"=w342, "Tabe"=w343, "Connncet State"=w344) -> ("error out"=w340:errorcluster, "state"=w339:bool)  [unwired: 2 in, 2 out]
        }
        n105 = Bundle By Name(cluster=w321, "mes.ProjectName"=w316, "mes.Line_Name"=w317, "mes.Shift"=w318, "mes.DateInfo"=w319, "Insert/Update(Run)"=w315) -> (w320:T12)
      }
      frame "Model:Get Actual & NG State(History)" {
        n106 = Unbundle By Name(w350) -> ("Main.Remote DB.Database"=w361:T6, "Mess FTT.Model"=w352:string, "Main.FTT TV"=w353:string, "Mode"=w345:enum16{"Eight", "EModel", "Outline"})
        n107 = call "Mes Class Time.vi"("error in (no error)"=w349, "Mode"=w345) -> ("error out"=w359:errorcluster, "Class"=w354:string, "s? t:f"=w355:timestamp)  [unwired: 6 in, 1 out]
        n108 = Format Date/Time String(time format string (%c)="%Y/%m/%d", seconds (now)=w355) -> (date/time string=w357:string)  [unwired: 1 in]
        n109 = for {
          tunnel: w361 -> [w375]
          tunnel: "Mes_History" -> [w374]
          tunnel: w352 -> [w373]
          tunnel: w357 -> [w368]
          tunnel: w354 -> [w367]
          tunnel: w353 -> [w366]
          tunnel: [w370] -> w351 mode=indexing
          shift-right: [w371] -> w348
          shift-left: w359 -> [w369]
          tunnel: string[] ["F1", "F2", "F3"] -> [w365] mode=indexing
          n110 = call "Mes Select Cmd.vi"("DateInfo"=w368, "h/r"=FALSE, "Shift"=w367, "Line_Name"=w366, "AvaType"=w365, "error in (no error)"=w369) -> ("resulting string"=w363:string, "error out"=w364:errorcluster)  [unwired: 8 in]
          n111 = call "DB Select data(Count index).vi"("index"=3, "Condtion"=w363, "error in (no error)"=w364, "Code"=w373, "Tabe"=w374, "Connncet State"=w375) -> ("error out"=w371:errorcluster, "state"=w370:bool)  [unwired: 2 in, 2 out]
        }
        n112 = Bundle By Name(cluster=w350, "Insert/Update(History)"=w351) -> (w347:T12)
      }
      frame "Model:Update Mes_Run" {
        n113 = Unbundle By Name(w388) -> ("Mess FTT.Model"=w386:string, "mes"=w401:T11, "Insert/Update(Run)"=w406:bool[], "Mess FTT.Actual"=w405:string, "Mess FTT.NG"=w404:string, "Main.Remote DB.Database"=w400:T6, "CT"=w377:string)
        n114 = Build Array(w405, w404, w377) -> (w403:string[])
        n115 = for {
          tunnel: w391 -> [w411]
          tunnel: w406 -> [w415] mode=indexing
          tunnel: w403 -> [w416]
          tunnel: string[] ["F1", "F2", "F3"] -> [w412] mode=indexing
          tunnel: w401 -> [w413]
          tunnel: w400 -> [w410]
          tunnel: "Mes_Run" -> [w409]
          tunnel: [w408] -> w398
          tunnel: [w407] -> w376 mode=indexing
          i -> [w417]
          n116 = Index Array(array=w416, index=w417) -> (element=w414:string)
          n117 = case shown="假" w415 {
            tunnel: w414 -> [w433 w456]
            tunnel: w413 -> [w435 w458]
            tunnel: w412 -> [w434 w457]
            tunnel: w411 -> [w432 w453]
            tunnel: w410 -> [w436 w455]
            tunnel: w409 -> [w430 w454]
            tunnel: [w437 w442] -> w408
            tunnel: [w421 w441] -> w407
            frame False {
              n118 = Bundle By Name(cluster=w435, "AvaType"=w434, "AvaValue"=w433) -> (w420:T11)
              n119 = Unbundle By Name(w420) -> ("DateInfo"=w427:timestamp, "Shift"=w424:string, "Line_Name"=w423:string, "AvaType"=w422:string)
              n120 = Format Date/Time String(time format string (%c)="%Y/%m/%d", seconds (now)=w427) -> (date/time string=w425:string)  [unwired: 1 in]
              n121 = call "Mes Select Cmd.vi"("DateInfo"=w425, "h/r"=TRUE, "Shift"=w424, "Line_Name"=w423, "AvaType"=w422, "error in (no error)"=w432) -> ("resulting string"=w428:string, "error out"=w431:errorcluster)  [unwired: 8 in]
              n122 = call "Mes Remote Table.vi"("mes"=w420) -> ("appended array"=w419:string[])  [unwired: 4 in]
              n123 = call "DB insert array data（Feedback).vi"("Condtion"=w428, "Data"=w419, "error in (no error)"=w431, "index"=3, "table"=w430, "Connncet State"=w436) -> ("error out"=w437:errorcluster, "state"=w421:bool)  [unwired: 3 in, 1 out]
            }
            frame True {
              n124 = Bundle By Name(cluster=w458, "AvaType"=w457, "AvaValue"=w456) -> (w451:T11)
              n125 = Unbundle By Name(w451) -> ("DateInfo"=w448:timestamp, "Shift"=w446:string, "Line_Name"=w445:string, "AvaType"=w444:string, "ProjectName"=w443:string)
              n126 = Format Date/Time String(time format string (%c)="%Y/%m/%d", seconds (now)=w448) -> (date/time string=w447:string)  [unwired: 1 in]
              n127 = call "Mes Select Cmd.vi"("DateInfo"=w447, "Shift"=w446, "Line_Name"=w445, "AvaType"=w444, "error in (no error)"=w453) -> ("resulting string"=w440:string, "error out"=w452:errorcluster)  [unwired: 9 in]
              n128 = To Variant(anything=w451) -> (Variant=w450:variant)
              n129 = call "DB Update Data(Feedback).vi"("Pos"=cluster{"index":i32, "Len":i32} {"index"=0, "Len"=7}, "condtinal"=w440, "Sel index"=3, "data"=w450, "error in (no error)"=w452, "Code"=w443, "table"=w454, "Connncet State"=w455) -> ("error out"=w442:errorcluster, "State"=w441:bool)  [unwired: 1 in, 1 out]
            }
          }
        }
        n130 = And Array Elements(Boolean array=w376) -> (logical AND=w392:bool)
        n131 = call "Error cyc Times.vi"("error in (no error)"=w398, "Status in"=w392) -> ("error out"=w390:errorcluster, "Numeric"=w383:i32, "Cys Status"=w397:bool, "Status out"=w395:bool)  [unwired: 6 in]
        n132 = Concatenate Strings("Model:" ("string"), w386, "-Mes实时表更新异常！" ("string")) -> (w394:string)
        n133 = Equal?(x=w383, y=2) -> (x = y?=w381:bool)
        n134 = Not(x=w395) -> (.not. x?=w396:bool)
        n135 = Select(t=string[] ["Model:Get Actual & NG", "Model:Update Mes_Run", "Display Tip"], s=w381, f=string[] ["Model:Get Actual & NG", "Model:Update Mes_Run"]) -> (s? t:f=w378:string[])
        n136 = Bundle By Name(cluster=w388, "information.cause"=w394, "information.Status"=w396) -> (w387:T12)
        n137 = Not(x=w397) -> (.not. x?=w385:bool)
      }
      frame "Model:Updata Mes_History" {
        n138 = Unbundle By Name(w462) -> ("mes"=w467:T11, "Insert/Update(History)"=w472:bool[], "Mess FTT.Actual"=w471:string, "Mess FTT.NG"=w470:string, "Main.Remote DB.Database"=w466:T6, "CT"=w464:string)
        n139 = Build Array(w471, w470, w464) -> (w469:string[])
        n140 = for {
          tunnel: w463 -> [w490]
          tunnel: w472 -> [w494] mode=indexing
          tunnel: w469 -> [w495]
          tunnel: string[] ["F1", "F2", "F3"] -> [w491] mode=indexing
          tunnel: w467 -> [w492]
          tunnel: w466 -> [w489]
          tunnel: "Mes_History" -> [w488]
          tunnel: [w487] -> w461
          tunnel: [w486] -> w459 mode=indexing
          i -> [w496]
          n141 = Index Array(array=w495, index=w496) -> (element=w493:string)
          n142 = case shown="假" w494 {
            tunnel: w493 -> [w512 w535]
            tunnel: w492 -> [w514 w537]
            tunnel: w491 -> [w513 w536]
            tunnel: w490 -> [w511 w532]
            tunnel: w489 -> [w515 w534]
            tunnel: w488 -> [w509 w533]
            tunnel: [w516 w521] -> w487
            tunnel: [w500 w520] -> w486
            frame False {
              n143 = Bundle By Name(cluster=w514, "AvaType"=w513, "AvaValue"=w512) -> (w499:T11)
              n144 = Unbundle By Name(w499) -> ("DateInfo"=w506:timestamp, "Shift"=w503:string, "Line_Name"=w502:string, "AvaType"=w501:string)
              n145 = Format Date/Time String(time format string (%c)="%Y/%m/%d", seconds (now)=w506) -> (date/time string=w504:string)  [unwired: 1 in]
              n146 = call "Mes Select Cmd.vi"("DateInfo"=w504, "h/r"=TRUE, "Shift"=w503, "Line_Name"=w502, "AvaType"=w501, "error in (no error)"=w511) -> ("resulting string"=w507:string, "error out"=w510:errorcluster)  [unwired: 8 in]
              n147 = call "Mes Remote Table.vi"("mes"=w499) -> ("appended array"=w498:string[])  [unwired: 4 in]
              n148 = call "DB insert array data（Feedback).vi"("Condtion"=w507, "Data"=w498, "error in (no error)"=w510, "index"=3, "table"=w509, "Connncet State"=w515) -> ("error out"=w516:errorcluster, "state"=w500:bool)  [unwired: 3 in, 1 out]
            }
            frame True {
              n149 = Bundle By Name(cluster=w537, "AvaType"=w536, "AvaValue"=w535) -> (w530:T11)
              n150 = Unbundle By Name(w530) -> ("DateInfo"=w527:timestamp, "Shift"=w525:string, "Line_Name"=w524:string, "AvaType"=w523:string, "ProjectName"=w522:string)
              n151 = Format Date/Time String(time format string (%c)="%Y/%m/%d", seconds (now)=w527) -> (date/time string=w526:string)  [unwired: 1 in]
              n152 = call "Mes Select Cmd.vi"("DateInfo"=w526, "Shift"=w525, "Line_Name"=w524, "AvaType"=w523, "error in (no error)"=w532) -> ("resulting string"=w519:string, "error out"=w531:errorcluster)  [unwired: 9 in]
              n153 = To Variant(anything=w530) -> (Variant=w529:variant)
              n154 = call "DB Update Data(Feedback).vi"("Pos"=cluster{"index":i32, "Len":i32} {"index"=0, "Len"=7}, "condtinal"=w519, "Sel index"=3, "data"=w529, "error in (no error)"=w531, "Code"=w522, "table"=w533, "Connncet State"=w534) -> ("error out"=w521:errorcluster, "State"=w520:bool)  [unwired: 1 in, 1 out]
            }
          }
        }
        n155 = And Array Elements(Boolean array=w459) -> (logical AND=w460:bool)
        n156 = call "Error cyc Times.vi"("error in (no error)"=w461, "Status in"=w460) -> ("error out"=w483:errorcluster, "Numeric"=w478:i32, "Cys Status"=w482:bool)  [unwired: 6 in, 1 out]
        n157 = Not(x=w482) -> (.not. x?=w481:bool)
        n158 = Equal?(x=w478, y=2) -> (x = y?=w476:bool)
        n159 = Bundle By Name(cluster=w462, "information.cause"="", "information.Status"=w481) -> (w480:T12)
        n160 = Select(t=string[] ["Model:Updata Mes_History", "Display Tip"], s=w476, f=string[] ["Model:Updata Mes_History"]) -> (s? t:f=w475:string[])
        n161 = Not(x=w482) -> (.not. x?=w484:bool)
      }
      frame "Model:Add Type" {
        n162 = Unbundle By Name(w552) -> ("Model"=w550:string[], "Mess FTT.Model"=w545:string, "Main.Path.Config"=w540:path)
        n163 = Search 1D Array(1D array=w550, element=w545) -> (index of element=w549:i32)  [unwired: 1 in]
        n164 = Greater Or Equal To 0?(x=w549) -> (x >= 0?=w548:bool)
        n165 = case shown="真" w548 {
          tunnel: [w556 w557] -> w539
          tunnel: w550 -> [w555 w557]
          tunnel: w545 -> [w554 _]
          frame False {
            n166 = Insert Into Array(array=w555, new element=w554) -> (w556:string[])  [unwired: 1 in]
          }
          frame True {
          }
        }
        n167 = Concatenate Strings("Model:" ("字符串"), w545, "Mes更新玩完成" ("字符串")) -> (w547:string)
        n168 = call "OP Model.vi"("error in (no error)"=w542, "Enum"=enum16{"init", "Read", "Write"}."Write", "ArrayStr"=w539, "Path"=w540) -> ("error out"=w541:errorcluster)  [unwired: 5 in, 2 out]
        n169 = Bundle By Name(cluster=w552, "Model"=w539, "information.cause"=w547, "information.Status"=FALSE) -> (w551:T12)
      }
      frame "Outline:Steps" {
        n170 = call "Special Time  UPH.vi"("error in (no error)"=w561) -> ("error out"=w559:errorcluster)  [unwired: 10 in]
        n171 = Wait (ms)(milliseconds to wait=u32 3000) -> ()  [unwired: 1 out]
        n172 = Unbundle By Name(w565) -> ("Model"=w563:string[])
        n173 = Bundle By Name(cluster=w565, "Outline_Type"=w563, "Mode"=enum16{"Eight", "EModel", "Outline"}."Outline") -> (w564:T12)
      }
      frame "Outline:Empty Type" {
        n174 = Unbundle By Name(w574) -> ()  [unwired: 1 out]
        n175 = call "Global Mes Triger.vi"("error in (no error)"=w572, "R/S"=FALSE) -> ("error out"=w571:errorcluster, "Var out"=w569:T15)  [unwired: 8 in]
        n176 = Unbundle By Name(w569) -> ("Model"=w568:string)
        n177 = Bundle By Name(cluster=w574, "Mess FTT.Model"=w568) -> (w573:T12)
        n178 = Empty String/Path?(string/path=w568) -> (empty?=w576:bool)
      }
      frame "Outline:Mes_Run Update" {
        n179 = Unbundle By Name(w584) -> ("Mess FTT.Model"=w591:string, "mes"=w600:T11, "Mess FTT.Actual"=w604:string, "Mess FTT.NG"=w603:string, "Main.Remote DB.Database"=w599:T6)  [unwired: 1 out]
        n180 = Build Array(w604, w603) -> (w602:string[])
        n181 = for {
          tunnel: w585 -> [w609]
          tunnel: bool[] [TRUE, TRUE] ("Insert/Update") -> [w613] mode=indexing
          tunnel: w602 -> [w614]
          tunnel: string[] ["F1", "F2"] -> [w610] mode=indexing
          tunnel: w600 -> [w611]
          tunnel: w599 -> [w608]
          tunnel: "Mes_Run" -> [w607]
          tunnel: [w606] -> w596
          tunnel: [w605] -> w597 mode=indexing
          i -> [w615]
          n182 = Index Array(array=w614, index=w615) -> (element=w612:string)
          n183 = case shown="假" w613 {
            tunnel: w612 -> [w631 w655]
            tunnel: w611 -> [w633 w657]
            tunnel: w610 -> [w632 w656]
            tunnel: w609 -> [w630 w652]
            tunnel: w608 -> [w634 w654]
            tunnel: w607 -> [w628 w653]
            tunnel: [w635 w641] -> w606
            tunnel: [w619 w640] -> w605
            frame False {
              n184 = Bundle By Name(cluster=w633, "AvaType"=w632, "AvaValue"=w631) -> (w618:T11)
              n185 = Unbundle By Name(w618) -> ("DateInfo"=w625:timestamp, "Shift"=w622:string, "Line_Name"=w621:string, "AvaType"=w620:string)
              n186 = Format Date/Time String(time format string (%c)="%Y/%m/%d", seconds (now)=w625) -> (date/time string=w623:string)  [unwired: 1 in]
              n187 = call "Mes Select Cmd.vi"("DateInfo"=w623, "h/r"=TRUE, "Shift"=w622, "Line_Name"=w621, "AvaType"=w620, "error in (no error)"=w630) -> ("resulting string"=w626:string, "error out"=w629:errorcluster)  [unwired: 8 in]
              n188 = call "Mes Remote Table.vi"("mes"=w618) -> ("appended array"=w617:string[])  [unwired: 4 in]
              n189 = call "DB insert array data（Feedback).vi"("Condtion"=w626, "Data"=w617, "error in (no error)"=w629, "index"=3, "table"=w628, "Connncet State"=w634) -> ("error out"=w635:errorcluster, "state"=w619:bool)  [unwired: 3 in, 1 out]
            }
            frame True {
              n190 = Bundle By Name(cluster=w657, "AvaType"=w656, "AvaValue"=w655) -> (w650:T11)
              n191 = Unbundle By Name(w650) -> ("DateInfo"=w647:timestamp, "Shift"=w645:string, "Line_Name"=w644:string, "AvaType"=w643:string, "ProjectName"=w642:string)
              n192 = Format Date/Time String(time format string (%c)="%Y/%m/%d", seconds (now)=w647) -> (date/time string=w646:string)  [unwired: 1 in]
              n193 = call "Mes Select Cmd.vi"("DateInfo"=w646, "h/r"=TRUE, "Shift"=w645, "Line_Name"=w644, "AvaType"=w643, "error in (no error)"=w652) -> ("resulting string"=w639:string, "error out"=w651:errorcluster)  [unwired: 8 in]
              n194 = To Variant(anything=w650) -> (Variant=w649:variant)
              n195 = call "DB Update Data(Feedback).vi"("Pos"=cluster{"index":i32, "Len":i32} {"index"=0, "Len"=7}, "condtinal"=w639, "Sel index"=3, "data"=w649, "error in (no error)"=w651, "Code"=w642, "table"=w653, "Connncet State"=w654) -> ("error out"=w641:errorcluster, "State"=w640:bool)  [unwired: 1 in, 1 out]
            }
          }
        }
        n196 = And Array Elements(Boolean array=w597) -> (logical AND=w588:bool)
        n197 = call "Error cyc Times.vi"("error in (no error)"=w596, "Status in"=w588) -> ("error out"=w582:errorcluster, "Cys Status"=w578:bool, "Status out"=w594:bool)  [unwired: 6 in, 1 out]
        n198 = Select(t="-下线Me实时表更新完成！" ("string"), s=w588, f="-下线Mes实时表更新异常！" ("string")) -> (s? t:f=w587:string)
        n199 = Concatenate Strings("Model:" ("string"), w591, w587) -> (w593:string)
        n200 = Not(x=w594) -> (.not. x?=w595:bool)
        n201 = Bundle By Name(cluster=w584, "information.cause"=w593, "information.Status"=w595) -> (w586:T12)
        n202 = Not(x=w578) -> (.not. x?=w579:bool)
      }
      frame "Outline:End Type Judge" {
        n203 = Unbundle By Name(w663) -> ("Outline_Type"=w667:string[])
        n204 = Delete From Array(array=w667, length=1, index=0) -> (array with subset deleted=w664:string[])  [unwired: 1 out]
        n205 = Empty Array?(array=w664) -> (empty?=w659:bool)
        n206 = Bundle By Name(cluster=w663, "Outline_Type"=w664) -> (w662:T12)
        n207 = Not(x=w659) -> (.not. x?=w658:bool)
      }
      frame "Complete Steps" {
        n208 = Bundle By Name(cluster=w675, "Mess FTT"=T9 {"Model"="", "Actual"="", "NG"=""}, "mes"=T11 {"DateInfo"=timestamp(0 s since 1904-01-01), "Shift"="", "Line_Name"="", "ProjectName"="", "AvaType"="", "AvaValue"="", "Remark"=""}, "Insert/Update(Run)"=bool[] [] ("Insert/Update")) -> (w674:T12)
      }
      frame "Input & Output" {
        n209 = Unbundle By Name(w682) -> ("Main.Ctr.Exit"=w679:refnum<vi>)
        n210 = property class="Bool (严格)"(reference=w679, error in=w680) -> (error out=w676:errorcluster, "Value"=w678:bool)  [unwired: 1 out]
      }
      frame "Quit" {
      }
      frame "Display Tip" {
        n211 = Unbundle By Name(w693) -> ("information"=w691:T10)
        n212 = Unbundle By Name(w689) -> ("source"=w688:string)
        n213 = Bundle By Name(cluster=w691, "Suroce"=w688) -> (w690:T10)
        n214 = call "Log info.vi"("error in (no error)"=w689, "information"=w690) -> ("error out"=w694:errorcluster)  [unwired: 8 in, 1 out]
      }
      frame "Error Log" {
        n215 = Unbundle By Name(w704) -> ("information"=w703:T10)
        n216 = Unbundle By Name(w697) -> ("source"=w696:string, "status"=w695:bool)
        n217 = Bundle By Name(cluster=w703, "Status"=TRUE, "Suroce"=w696, "Status"=w695) -> (w702:T10)
        n218 = call "Log info.vi"("error in (no error)"=w697, "information"=w702) -> ("error out"=w706:errorcluster)  [unwired: 8 in, 1 out]
        n219 = call <vilib>:"Clear Errors.vi"("error in (no error)"=w706) -> ("error out"=w705:errorcluster)  [unwired: 5 in, 1 out]
      }
    }
    n220 = call "Insert Multiple Events(Error).vi"("error in (no error)"=w17, "Insert all? (T)"=w21, "Events to Insert"=w20, "Event queue in"=w22) -> ("error out"=w16:errorcluster, "Event queue out"=w23:string[])  [unwired: 6 in]
  }
  "error out" <- w9
